vi "next chunk - V4.vi"(7 "next chunk action":T1=enum."", 9 "x + iy":cdb[](array[numeric])=[0.0014961444378751654-0.005494848789731022i, 0.0014279223595474386-0.005470747752736027i, 0.001513711413730512-0.00552874878044623i, 0.001502407562898675-0.005445638194888334i, 0.0015845696982058808-0.005437153149732619i, 0.0015101628497750257-0.005522728337901211i, 0.0015131031857027845-0.005520920485579818i, 0.0015751707865244427-0.005432155579139866i, 0.001381283887581937-0.0055376532176146485i, 0.0013869914972504977-0.005471269712968517i], 10 "chunks":T2={"start F (Hz)"=300000.0, "stop F (Hz)"=600000.0, "total number of points"=3000, "chunk size"=10, "freq step (Hz)"=0.0, "update rate (Hz)"=0.0, "adaptive parameters"={"peaks are known -- parameters"={"Def Gamma (kHz)"=0.5, "dV"=17.0, "time in Gamma (sec)"=7.0, "phi-star"=0.0, "all peaks (kHz)"=[], "delta t (sec)"=22.0, "default step (Hz)"=0.0, "all gamma (kHz)"=[564.0, 649.0, 987.0, 1133.0, 1214.0, 1585.0, 1763.0, 1823.0, 1880.0, 1899.0, 2032.0, 2138.0, 2221.0, 2270.0, 2350.0, 2456.0, 2580.0, 2634.0, 2831.0, 2960.0, 2965.0, 3131.0, 3328.0, 3469.0, 3553.0, 0.0, 3615.0, 3734.0, 0.0, 0.0, 0.0, 4236.0, 4300.0, 4331.0], "peaks OK"=FALSE, "gamma OK"=FALSE, "near omega (kHz)"=0.0, "near gamma (kHz)"=0.0, "min step (Hz)"=10000.0, "max step(Hz)"=0.01, "min gamma (kHz)"=0.01, "all time in gamma (sec)"=[], "time in gamma OK"=FALSE, "time-in-gamma mode"=enum."same for all"}, "find peak - parameters"={"wavepacket"={"R"=0.5, "wave number"=17.0, "delta k"=7.0, "radii vector"=[], "radial section"=[], "wave vector"=22.0, "wavepacket is"=TRUE}, "number of grid points"=70, "decimation threshold"=1, "Voltage range"=0.1, "target freq step"=20.0, "target spot size"=0.05, "factor"=1.0, "another factor"=1.0, "analyze last # sec"=3, "scale factor"=3}}, "total sweep time (sec)"=0.0, "chunk time (sec)"=0.0, "spot size (V)"=0.0, "uniform freq step (Hz)"=0.0, "next start freq (Hz)"=0.0} {"next start freq (Hz)" format="%#9_8f"; "uniform freq step (Hz)" format="%#_3f"; "spot size (V)" format="%#_2f"; "adaptive parameters"."find peak - parameters"."wavepacket"."delta k" format="%#_3f"; "adaptive parameters"."find peak - parameters"."wavepacket"."wave number" format="%#_3f"; "adaptive parameters"."find peak - parameters"."wavepacket"."R" format="%#_3f"; "freq step (Hz)" format="%#4_4f"; "stop F (Hz)" format="%#_3f"; "start F (Hz)" format="%#_3f"}, 11 "F Array in":dbl[](array[numeric])) -> (2 "chunks out":T2={"start F (Hz)"=1400000.0, "stop F (Hz)"=3000000.0, "total number of points"=6000, "chunk size"=10, "freq step (Hz)"=400.0, "update rate (Hz)"=250.0, "adaptive parameters"={"peaks are known -- parameters"={"Def Gamma (kHz)"=0.5, "dV"=17.0, "time in Gamma (sec)"=7.0, "phi-star"=0.0, "all peaks (kHz)"=[], "delta t (sec)"=22.0, "default step (Hz)"=0.0, "all gamma (kHz)"=[564.0, 649.0, 987.0, 1133.0, 1214.0, 1585.0, 1763.0, 1823.0, 1880.0, 1899.0, 2032.0, 2138.0, 2221.0, 2270.0, 2350.0, 2456.0, 2580.0, 2634.0, 2831.0, 2960.0, 2965.0, 3131.0, 3328.0, 3469.0, 3553.0, 0.0, 3615.0, 3734.0, 0.0, 0.0, 0.0, 4236.0, 4300.0, 4331.0], "peaks OK"=FALSE, "gamma OK"=FALSE, "near omega (kHz)"=0.0, "near gamma (kHz)"=0.0, "min step (Hz)"=10000.0, "max step(Hz)"=0.01, "min gamma (kHz)"=0.01, "all time in gamma (sec)"=[], "time in gamma OK"=FALSE, "time-in-gamma mode"=enum."same for all"}, "find peak - parameters"={"wavepacket"={"R"=0.5, "wave number"=17.0, "delta k"=7.0, "radii vector"=[], "radial section"=[], "wave vector"=22.0, "wavepacket is"=TRUE}, "number of grid points"=70, "decimation threshold"=1, "Voltage range"=0.1, "target freq step"=20.0, "target spot size"=0.05, "factor"=1.0, "another factor"=1.0, "analyze last # sec"=3, "scale factor"=3}}, "total sweep time (sec)"=24.0, "chunk time (sec)"=0.04, "spot size (V)"=5.8152639158694506e-05, "uniform freq step (Hz)"=266.6666666666667, "next start freq (Hz)"=1412960.0000000002} {"next start freq (Hz)" format="%#9_8f"; "uniform freq step (Hz)" format="%#_3f"; "spot size (V)" format="%#_2f"; "adaptive parameters"."find peak - parameters"."wavepacket"."delta k" format="%#_3f"; "adaptive parameters"."find peak - parameters"."wavepacket"."wave number" format="%#_3f"; "adaptive parameters"."find peak - parameters"."wavepacket"."R" format="%#_3f"; "freq step (Hz)" format="%#4_4f"; "stop F (Hz)" format="%#_3f"; "start F (Hz)" format="%#_3f"}, 3 "F Array out":dbl[](array[numeric]), 4 "fancy lines":cluster{dbl[], dbl[]}[](array[cluster])=[{[0.004347976639836461, 0.0043237329011621035, 0.004251384023380436, 0.004132070991513198, 0.003967675443347089, 0.0037607899948818246, 0.0035146773532270816, 0.00323321886176232, 0.0029208532890330928, 0.002582506826719488, 0.00222351540065057, 0.0018495405200665291, 0.0014664799922359413, 0.001080374910511962, 0.0006973143826813736, 0.0003233395020973332, -3.56519239715844e-05, -0.0003739983862851902, -0.0006863639590144167, -0.0009678224504791784, -0.0012139350921339205, -0.0014208205405991845, -0.001585216088765295, -0.0017045291206325324, -0.0017768779984142003, -0.001801121737088557, -0.0017768779984142003, -0.0017045291206325324, -0.0015852160887652941, -0.001420820540599184, -0.00121393509213392, -0.000967822450479178, -0.0006863639590144162, -0.00037399838628518847, -3.5651923971582664e-05, 0.0003233395020973332, 0.0006973143826813741, 0.0010803749105119625, 0.0014664799922359426, 0.001849540520066531, 0.0022235154006505697, 0.002582506826719488, 0.0029208532890330936, 0.003233218861762321, 0.003514677353227083, 0.0037607899948818254, 0.003967675443347089, 0.004132070991513199, 0.004251384023380437, 0.0043237329011621035], [-0.00253283204245687, -0.0021474888509143563, -0.001768222751695333, -0.0014010149977470693, -0.0010516566747086093, -0.0007256573720308159, -0.00042815829345946126, -0.00016385117718095135, 6.309569569158376e-05, 0.0002491032374014545, 0.0003912379979003752, 0.0004872584271080889, 0.0005356502254961651, 0.0005356502254961651, 0.00048725842710808844, 0.0003912379979003752, 0.00024910323740145405, 6.309569569158376e-05, -0.00016385117718095135, -0.0004281582934594617, -0.0007256573720308154, -0.0010516566747086097, -0.00140101499774707, -0.0017682227516953328, -0.0021474888509143567, -0.002532832042456871, -0.002918175233999384, -0.003297441333218408, -0.003664649087166672, -0.004014007410205131, -0.004340006712882925, -0.004637505791454279, -0.004901812907732789, -0.005128759780605325, -0.005314767322315195, -0.005456902082814115, -0.0055529225120218295, -0.005601314310409906, -0.005601314310409906, -0.005552922512021829, -0.005456902082814115, -0.005314767322315195, -0.0051287597806053235, -0.004901812907732788, -0.004637505791454277, -0.004340006712882922, -0.004014007410205131, -0.0036646490871666704, -0.0032974413332184063, -0.0029181752339993822]}, {[-0.0007985969840225416, -0.0005913945404828922, -0.0003841920969432428, -0.0001769896534035934, 3.0212790136055923e-05, 0.00023741523367570524, 0.0004446176772153548, 0.0006518201207550041, 0.0008590225642946534, 0.0010662250078343027, 0.001273427451373952, 0.0014806298949136016, 0.001687832338453251, 0.0018950347819929002, 0.00210223722553255, 0.0023094396690721986, 0.002516642112611848, 0.0027238445561514977, 0.0029310469996911472, 0.003138249443230796], [-0.004804300169328853, -0.004577153356641655, -0.004350006543954456, -0.004122859731267258, -0.00389571291858006, -0.0036685661058928616, -0.003441419293205663, -0.003214272480518465, -0.0029871256678312666, -0.002759978855144068, -0.00253283204245687, -0.0023056852297696716, -0.002078538417082473, -0.0018513916043952751, -0.0016242447917080766, -0.0013970979790208786, -0.0011699511663336801, -0.0009428043536464817, -0.0007156575409592832, -0.0004885107282720852]}, {[-0.0009980406754980312, -0.0007708938628108329, -0.0005437470501236345, -0.0003166002374364362, -8.945342474923792e-05, 0.00013769338793796033, 0.0003648402006251588, 0.0005919870133123571, 0.0008191338259995553, 0.0010462806386867538, 0.0012734274513739518, 0.0015005742640611503, 0.0017277210767483488, 0.001954867889435547, 0.0021820147021227453, 0.0024091615148099433, 0.002636308327497142, 0.0028634551401843403, 0.0030906019528715387, 0.0033177487655587368], [-0.0004608076070603765, -0.0006680100506000258, -0.0008752124941396752, -0.0010824149376793247, -0.001289617381218974, -0.0014968198247586233, -0.0017040222682982728, -0.0019112247118379222, -0.0021184271553775715, -0.0023256295989172206, -0.00253283204245687, -0.0027400344859965196, -0.002947236929536169, -0.0031544393730758183, -0.003361641816615468, -0.003568844260155117, -0.0037760467036947664, -0.003983249147234416, -0.004190451590774065, -0.004397654034313714]}], 6 "fancy circles":cluster{dbl[], dbl[]}[](array[cluster])=[{[0.004347976639836461, 0.0043237329011621035, 0.004251384023380436, 0.004132070991513198, 0.003967675443347089, 0.0037607899948818246, 0.0035146773532270816, 0.00323321886176232, 0.0029208532890330928, 0.002582506826719488, 0.00222351540065057, 0.0018495405200665291, 0.0014664799922359413, 0.001080374910511962, 0.0006973143826813736, 0.0003233395020973332, -3.56519239715844e-05, -0.0003739983862851902, -0.0006863639590144167, -0.0009678224504791784, -0.0012139350921339205, -0.0014208205405991845, -0.001585216088765295, -0.0017045291206325324, -0.0017768779984142003, -0.001801121737088557, -0.0017768779984142003, -0.0017045291206325324, -0.0015852160887652941, -0.001420820540599184, -0.00121393509213392, -0.000967822450479178, -0.0006863639590144162, -0.00037399838628518847, -3.5651923971582664e-05, 0.0003233395020973332, 0.0006973143826813741, 0.0010803749105119625, 0.0014664799922359426, 0.001849540520066531, 0.0022235154006505697, 0.002582506826719488, 0.0029208532890330936, 0.003233218861762321, 0.003514677353227083, 0.0037607899948818254, 0.003967675443347089, 0.004132070991513199, 0.004251384023380437, 0.0043237329011621035], [-0.00253283204245687, -0.0021474888509143563, -0.001768222751695333, -0.0014010149977470693, -0.0010516566747086093, -0.0007256573720308159, -0.00042815829345946126, -0.00016385117718095135, 6.309569569158376e-05, 0.0002491032374014545, 0.0003912379979003752, 0.0004872584271080889, 0.0005356502254961651, 0.0005356502254961651, 0.00048725842710808844, 0.0003912379979003752, 0.00024910323740145405, 6.309569569158376e-05, -0.00016385117718095135, -0.0004281582934594617, -0.0007256573720308154, -0.0010516566747086097, -0.00140101499774707, -0.0017682227516953328, -0.0021474888509143567, -0.002532832042456871, -0.002918175233999384, -0.003297441333218408, -0.003664649087166672, -0.004014007410205131, -0.004340006712882925, -0.004637505791454279, -0.004901812907732789, -0.005128759780605325, -0.005314767322315195, -0.005456902082814115, -0.0055529225120218295, -0.005601314310409906, -0.005601314310409906, -0.005552922512021829, -0.005456902082814115, -0.005314767322315195, -0.0051287597806053235, -0.004901812907732788, -0.004637505791454277, -0.004340006712882922, -0.004014007410205131, -0.0036646490871666704, -0.0032974413332184063, -0.0029181752339993822]}, {[-0.0007985969840225416, -0.0005913945404828922, -0.0003841920969432428, -0.0001769896534035934, 3.0212790136055923e-05, 0.00023741523367570524, 0.0004446176772153548, 0.0006518201207550041, 0.0008590225642946534, 0.0010662250078343027, 0.001273427451373952, 0.0014806298949136016, 0.001687832338453251, 0.0018950347819929002, 0.00210223722553255, 0.0023094396690721986, 0.002516642112611848, 0.0027238445561514977, 0.0029310469996911472, 0.003138249443230796], [-0.004804300169328853, -0.004577153356641655, -0.004350006543954456, -0.004122859731267258, -0.00389571291858006, -0.0036685661058928616, -0.003441419293205663, -0.003214272480518465, -0.0029871256678312666, -0.002759978855144068, -0.00253283204245687, -0.0023056852297696716, -0.002078538417082473, -0.0018513916043952751, -0.0016242447917080766, -0.0013970979790208786, -0.0011699511663336801, -0.0009428043536464817, -0.0007156575409592832, -0.0004885107282720852]}, {[-0.0009980406754980312, -0.0007708938628108329, -0.0005437470501236345, -0.0003166002374364362, -8.945342474923792e-05, 0.00013769338793796033, 0.0003648402006251588, 0.0005919870133123571, 0.0008191338259995553, 0.0010462806386867538, 0.0012734274513739518, 0.0015005742640611503, 0.0017277210767483488, 0.001954867889435547, 0.0021820147021227453, 0.0024091615148099433, 0.002636308327497142, 0.0028634551401843403, 0.0030906019528715387, 0.0033177487655587368], [-0.0004608076070603765, -0.0006680100506000258, -0.0008752124941396752, -0.0010824149376793247, -0.001289617381218974, -0.0014968198247586233, -0.0017040222682982728, -0.0019112247118379222, -0.0021184271553775715, -0.0023256295989172206, -0.00253283204245687, -0.0027400344859965196, -0.002947236929536169, -0.0031544393730758183, -0.003361641816615468, -0.003568844260155117, -0.0037760467036947664, -0.003983249147234416, -0.004190451590774065, -0.004397654034313714]}])   [LabVIEW 2015]
uses:
  single sweep - frequency chunks.ctl
  single sweep - adaptive parameters.ctl
  next chunk -- parameters.ctl
  time in gamma mode control.ctl
  find peak -- parameters.ctl
  wavepacket.ctl
  next chunk -- action.ctl
  stack action -- control.ctl
  Q -- check range -- i -- real.vi
  array -- find interval - real.vi
  trig -- arctan.vi
  Q - not nan -- real.vi
panel:
  in  "to":dbl=0.001
  in  "from":dbl=-0.001
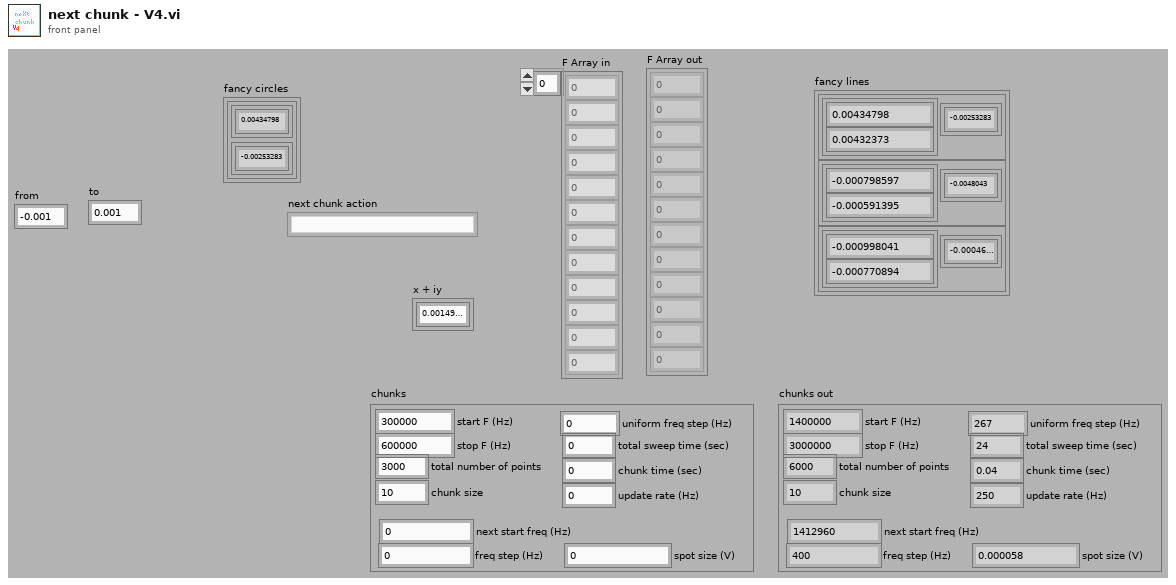
[diagram p1: front panel]
types:
  T1 = typedef "next chunk -- action.ctl" = enum16{"empty", "init - uniform", "next chunk - uniform", "next chunk - peaks are known", "init - peaks are known", ""}
  T2 = typedef "single sweep - frequency chunks.ctl" = cluster{"start F (Hz)":dbl, "stop F (Hz)":dbl, "total number of points":i32, "chunk size":i32, "freq step (Hz)":dbl, "update rate (Hz)":dbl, "adaptive parameters":T3, "total sweep time (sec)":dbl, "chunk time (sec)":dbl, "spot size (V)":dbl, "uniform freq step (Hz)":dbl, "next start freq (Hz)":dbl}
  T3 = typedef "single sweep - adaptive parameters.ctl" = cluster{"peaks are known -- parameters":T4, "find peak - parameters":T6}
  T4 = typedef "next chunk -- parameters.ctl" = cluster{"Def Gamma (kHz)":dbl, "dV":dbl, "time in Gamma (sec)":dbl, "phi-star":dbl, "all peaks (kHz)":dbl[], "delta t (sec)":dbl, "default step (Hz)":dbl, "all gamma (kHz)":dbl[], "peaks OK":bool, "gamma OK":bool, "near omega (kHz)":dbl, "near gamma (kHz)":dbl, "min step (Hz)":dbl, "max step(Hz)":dbl, "min gamma (kHz)":dbl, "all time in gamma (sec)":dbl[], "time in gamma OK":bool, "time-in-gamma mode":T5}
  T5 = typedef "time in gamma mode control.ctl" = enum16{"same for all", "each one different", "uniform scan"}
  T6 = typedef "find peak -- parameters.ctl" = cluster{"wavepacket":T7, "number of grid points":i32, "decimation threshold":i32, "Voltage range":dbl, "target freq step":dbl, "target spot size":dbl, "factor":dbl, "another factor":dbl, "analyze last # sec":i32, "scale factor":i32}
  T7 = typedef "wavepacket.ctl" = cluster{"R":dbl, "wave number":dbl, "delta k":dbl, "radii vector":dbl[], "radial section":cdb[], "wave vector":dbl, "wavepacket is":bool}
  T8 = cluster{"frequency step (Hz)":dbl, "next start frequency (Hz)":dbl, "number of chunks so far":i32, "chunk size":i32, "chunk time (sec)":dbl}
  T9 = typedef "stack action -- control.ctl" = enum16{"push", "pop", "check", "init"}
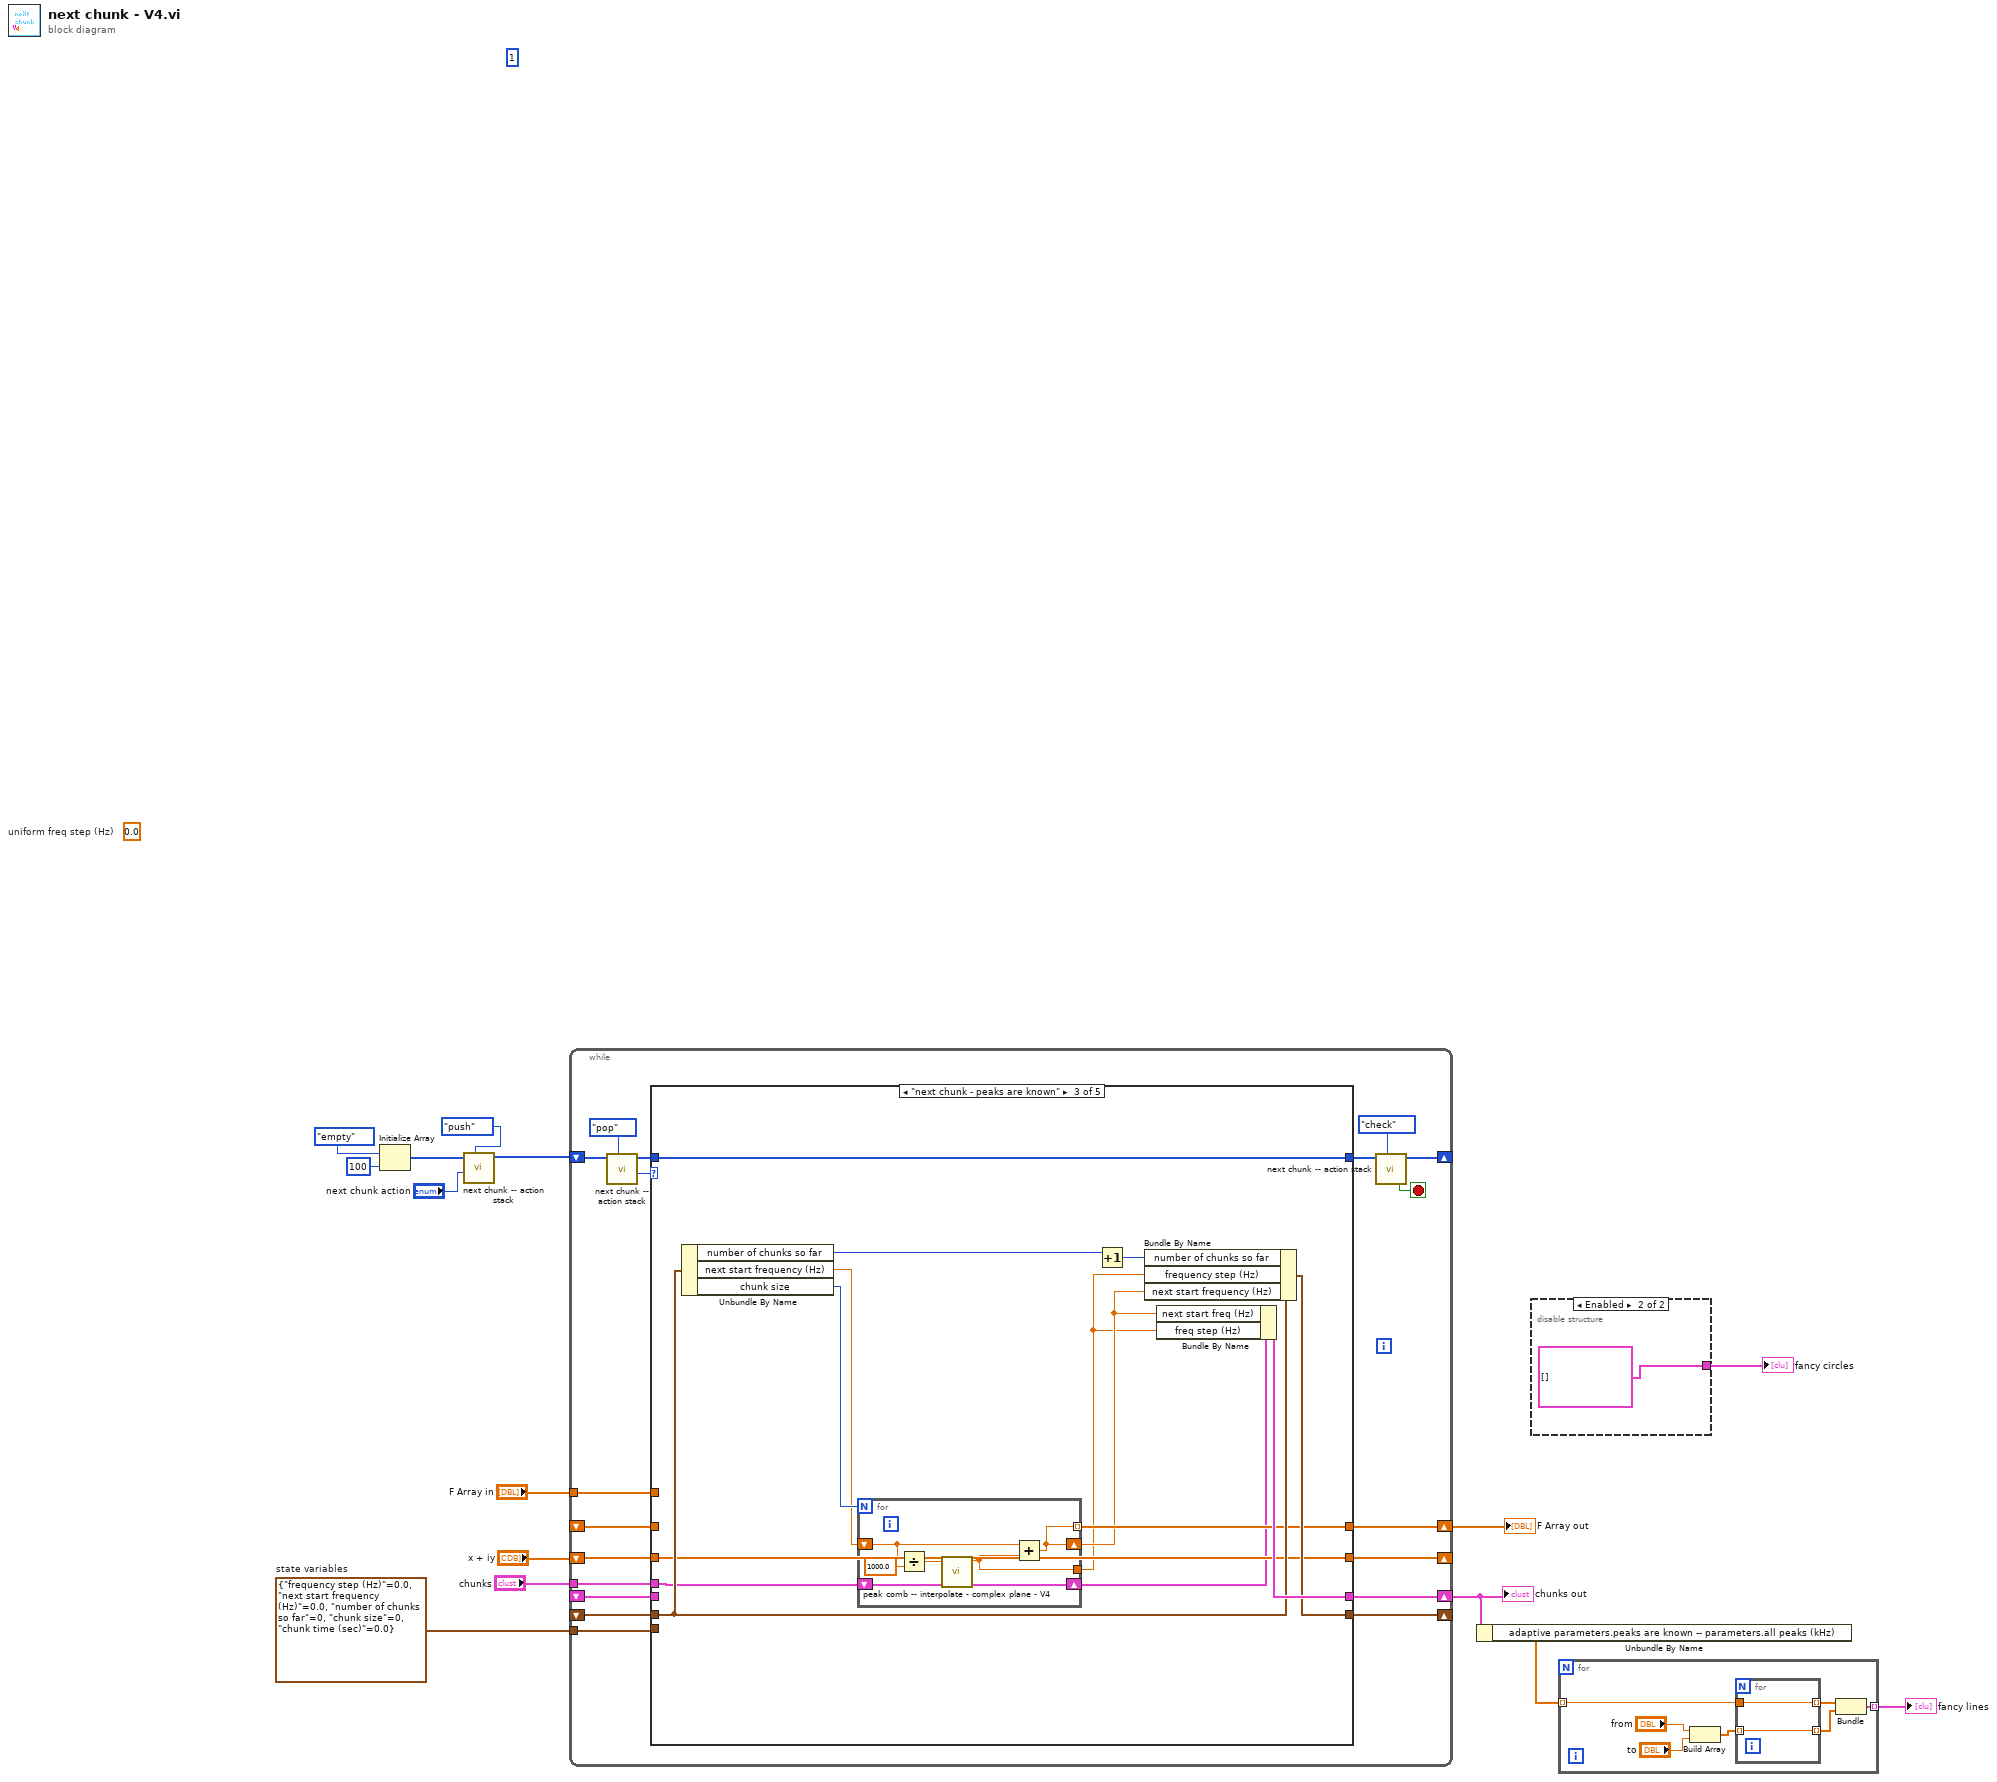
[diagram p0: block diagram]
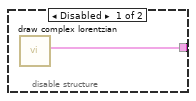
[diagram p2: hidden frame]
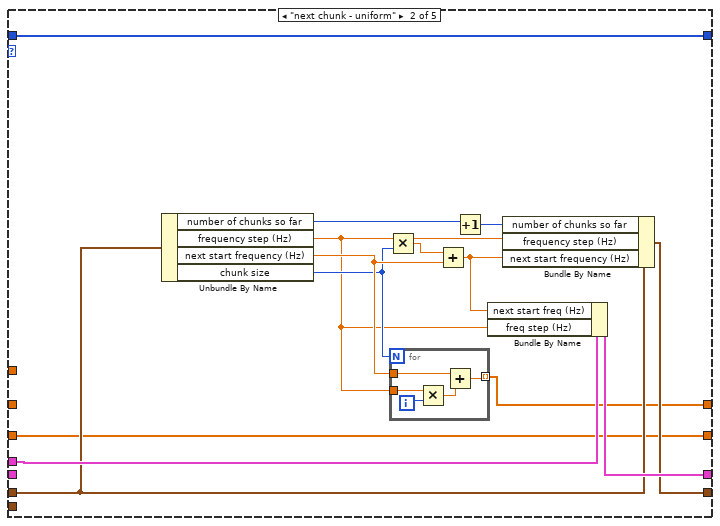
[diagram p4: hidden frame]
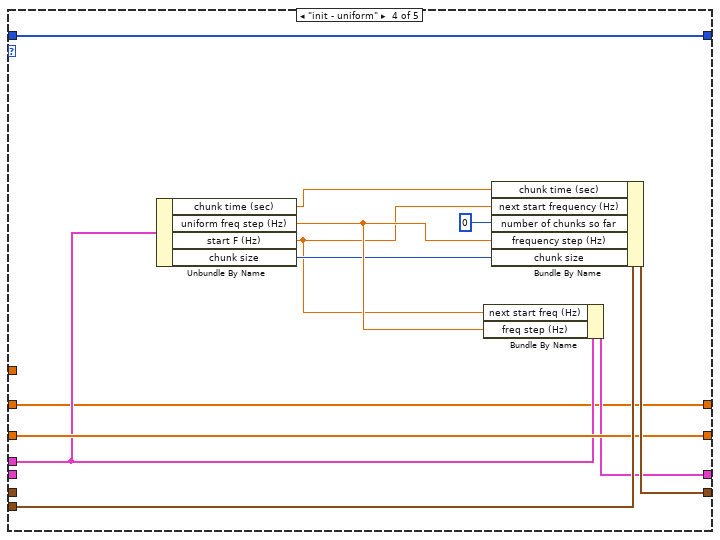
[diagram p5: hidden frame]
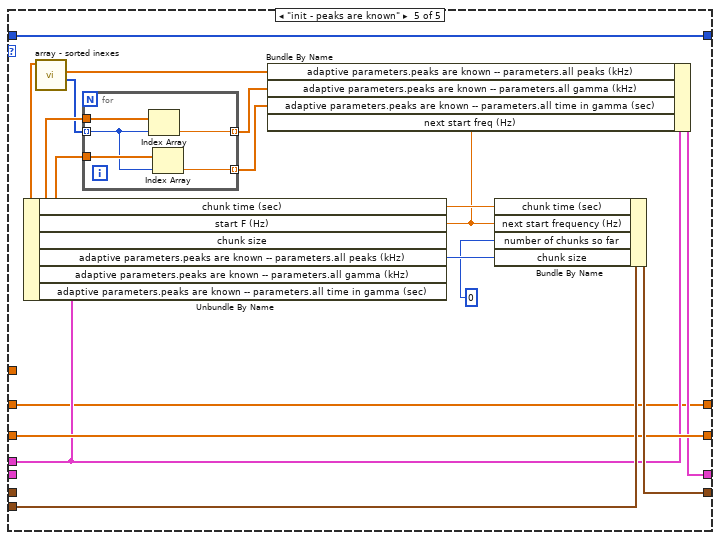
[diagram p6: hidden frame]
diagram:
  w10 = T8 {"frequency step (Hz)"=0.0, "next start frequency (Hz)"=0.0, "number of chunks so far"=0, "chunk size"=0, "chunk time (sec)"=0.0}  # state variables
  (unwired) 0.0  # uniform freq step (Hz)
  (unwired) 1
  n1 = Initialize Array(next_chunk_--_action."empty" ("next chunk action"), 100 ("dimension size")) -> (w4:T1[])
  n2 = call "next chunk -- action stack.vi"("stack action"=stack_action_--_control."push", "next chunk action"="next chunk action", "command stack"=w4) -> ("command stack out"=w3:T1[])  [unwired: 6 in, 2 out]
  n3 = while {
    shift-right: [w29] -> _
    shift-left: w3 -> [w34]
    shift-right: [w26] -> _
    shift-left: _ -> [w25]
    shift-right: [w24] -> w5
    shift-left: _ -> [w23]
    shift-right: [w22] -> w7
    shift-left: _ -> [w21]
    shift-right: [w20] -> _
    shift-left: "x + iy" -> [w19]
    tunnel: "F Array in" -> [w18]
    tunnel: w10 -> [w17]
    tunnel: "chunks" -> [w16]
    stop <- w28 stop-if-true
    n4 = call "next chunk -- action stack.vi"("stack action"=stack_action_--_control."pop", "command stack"=w34) -> ("next chunk action out"=w27:T1, "command stack out"=w32:T1[])  [unwired: 7 in, 1 out]
    n5 = case shown="\"next chunk - peaks are known\"" w27 {
      tunnel: [w39 w47 w67 w91 w109] -> w30
      tunnel: w32 -> [w39 w47 w67 w91 w109]
      tunnel: [w38 w51 w71 w89 w107] -> w26
      tunnel: w25 -> [w38 w50 w70 _ _]
      tunnel: [w37 w52 w72 w86 w104] -> w24
      tunnel: w23 -> [w37 _ _ _ _]
      tunnel: [w36 w49 w69 w82 w101] -> w22
      tunnel: w21 -> [w36 _ _ w82 w101]
      tunnel: w19 -> [w35 w48 w68 w88 w106]
      tunnel: [w35 w48 w68 w88 w106] -> w20
      tunnel: w18 -> [_ _ _ _ _]
      tunnel: w17 -> [_ _ _ w90 w108]
      tunnel: w16 -> [_ w53 w60 w87 w105]
      frame "empty", Default {
      }
      frame "next chunk - uniform" {
        n6 = Unbundle By Name(w50) -> ("number of chunks so far"=w40:i32, "frequency step (Hz)"=w43:dbl, "next start frequency (Hz)"=w45:dbl, "chunk size"=w44:i32)
        n7 = Multiply(x=w43, y=w44) -> (x*y=w46:dbl)
        n8 = for {
          N: w44 -> [_]
          tunnel: w43 -> [w58]
          tunnel: [w56] -> w49 mode=indexing
          tunnel: w45 -> [w54]
          i -> [w55]
          n9 = Multiply(x=w58, y=w55) -> (x*y=w57:dbl)
          n10 = Add(x=w54, y=w57) -> (x+y=w56:dbl)
        }
        n11 = Add(x=w46, y=w45) -> (x+y=w41:dbl)
        n12 = Increment(x=w40) -> (x+1=w42:i32)
        n13 = Bundle By Name(cluster=w53, "next start freq (Hz)"=w41, "freq step (Hz)"=w43) -> (w52:T2)
        n14 = Bundle By Name(cluster=w50, "number of chunks so far"=w42, "frequency step (Hz)"=w43, "next start frequency (Hz)"=w41) -> (w51:T8)
      }
      frame "next chunk - peaks are known" {
        n15 = Unbundle By Name(w70) -> ("number of chunks so far"=w64:i32, "next start frequency (Hz)"=w63:dbl, "chunk size"=w66:i32)
        n16 = for {
          N: w66 -> [_]
          tunnel: [w76] -> w69 mode=indexing
          shift-right: [w76] -> w62
          shift-left: w63 -> [w77]
          tunnel: [w75] -> w61
          shift-right: [w73] -> w59
          shift-left: w60 -> [w74]
          n17 = Divide(x=w77, y=1000.0) -> (x/y=w79:dbl)
          n18 = call "peak comb -- interpolate - complex plane - V4.vi"("chunks"=w74, "freq (kHz)"=w79) -> ("chunks OUT"=w73:T2, "delta-F (Hz)"=w75:dbl)  [unwired: 6 in, 2 out]
          n19 = Add(x=w77, y=w75) -> (x+y=w76:dbl)
        }
        n20 = Increment(x=w64) -> (x+1=w65:i32)
        n21 = Bundle By Name(cluster=w70, "number of chunks so far"=w65, "frequency step (Hz)"=w61, "next start frequency (Hz)"=w62) -> (w71:T8)
        n22 = Bundle By Name(cluster=w59, "next start freq (Hz)"=w62, "freq step (Hz)"=w61) -> (w72:T2)
      }
      frame "init - uniform" {
        n23 = Unbundle By Name(w87) -> ("chunk time (sec)"=w83:dbl, "uniform freq step (Hz)"=w85:dbl, "start F (Hz)"=w81:dbl, "chunk size"=w84:i32)
        n24 = Bundle By Name(cluster=w87, "next start freq (Hz)"=w81, "freq step (Hz)"=w85) -> (w86:T2)
        n25 = Bundle By Name(cluster=w90, "chunk time (sec)"=w83, "next start frequency (Hz)"=w81, "number of chunks so far"=0, "frequency step (Hz)"=w85, "chunk size"=w84) -> (w89:T8)
      }
      frame "init - peaks are known" {
        n26 = Unbundle By Name(w105) -> ("chunk time (sec)"=w102:dbl, "start F (Hz)"=w99:dbl, "chunk size"=w103:i32, "adaptive parameters.peaks are known -- parameters.all peaks (kHz)"=w98:dbl[], "adaptive parameters.peaks are known -- parameters.all gamma (kHz)"=w96:dbl[], "adaptive parameters.peaks are known -- parameters.all time in gamma (sec)"=w93:dbl[])
        n27 = call "array - sorted inexes.vi"("x"=w98) -> ("index array"=w95:i32[], "sorted array"=w97:dbl[])  [unwired: 9 in]
        n28 = for {
          tunnel: w96 -> [w114]
          tunnel: w95 -> [w111] mode=indexing
          tunnel: [w113] -> w94 mode=indexing
          tunnel: w93 -> [w112]
          tunnel: [w110] -> w92 mode=indexing
          n29 = Index Array(array=w114, index=w111) -> (element=w113:dbl)
          n30 = Index Array(array=w112, index=w111) -> (element=w110:dbl)
        }
        n31 = Bundle By Name(cluster=w105, "adaptive parameters.peaks are known -- parameters.all peaks (kHz)"=w97, "adaptive parameters.peaks are known -- parameters.all gamma (kHz)"=w94, "adaptive parameters.peaks are known -- parameters.all time in gamma (sec)"=w92, "next start freq (Hz)"=w99) -> (w104:T2)
        n32 = Bundle By Name(cluster=w108, "chunk time (sec)"=w102, "next start frequency (Hz)"=w99, "number of chunks so far"=0, "chunk size"=w103) -> (w107:T8)
      }
    }
    n33 = call "next chunk -- action stack.vi"("stack action"=stack_action_--_control."check", "command stack"=w30) -> ("stack is empty ?"=w28:bool, "command stack out"=w29:T1[])  [unwired: 7 in, 1 out]
  }
  "F Array out" <- w7
  "chunks out" <- w5
  n34 = Unbundle By Name(w5) -> ("adaptive parameters.peaks are known -- parameters.all peaks (kHz)"=w1:dbl[])
  n35 = disable-structure shown="Enabled" {
    disable-tunnel: [w115 cluster{dbl[], dbl[]}[] [] ("fancy circles 2")] -> w6
    frame Disabled {
      n36 = call "draw complex lorentzian.vi"() -> ("fancy circles"=w115:cluster{dbl[], dbl[]}[])  [unwired: 11 in]
    }
    frame Enabled {
    }
  }
  "fancy circles" <- w6
  n37 = for {
    tunnel: w1 -> [w119] mode=indexing
    tunnel: [w117] -> w2 mode=indexing
    n38 = Build Array("from", "to") -> (w121:dbl[])
    n39 = for {
      tunnel: w121 -> [w125] mode=indexing
      tunnel: [w125] -> w120 mode=indexing
      tunnel: w119 -> [w124]
      tunnel: [w124] -> w118 mode=indexing
    }
    n40 = Bundle(w118, w120) -> (w117:cluster{dbl[], dbl[]})  [unwired: 1 in]
  }
  "fancy lines" <- w2
